vi "Configure Adjacent Channel Power (Measurement Setup).vi"(0 "VISA resource name":refnum<visa-resource-name>, 5 "ACP Carrier Number (1)":i32=1 min=1, 7 "ACP Measurement Method (0:Mod)":i32(ring) items=["Mod", "Total Power", "Inband Channel Bandwidth", "Both Sides", "Number"], 9 "ACP Display Type (0:Carrier)":i32(ring) items=["Carrier", "Offset Channel", "All"], 11 "error in (no error)":errorcluster) -> (4 "VISA resource name out":refnum<visa-resource-name>, 15 "error out":errorcluster)   [LabVIEW 2020, in "Anritsu Signal Analyzer Series.lvlib"]
doc: "Configures the ACP measurement parameters settings of the spectrum analyzer."
uses:
  Anritsu Signal Analyzer Series.lvlib
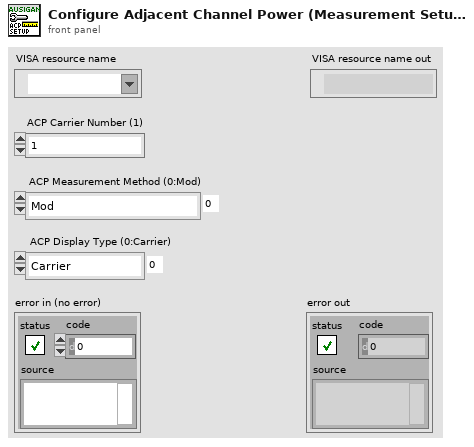
[diagram p1: front panel]
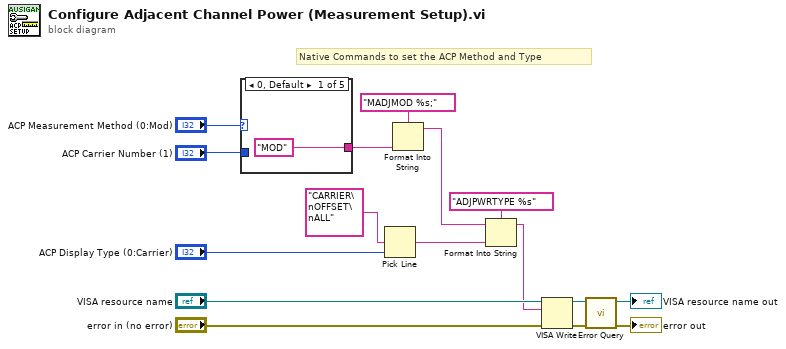
[diagram p0: block diagram]
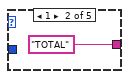
[diagram p2: hidden frame]
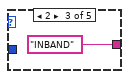
[diagram p3: hidden frame]
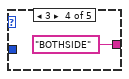
[diagram p4: hidden frame]
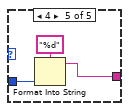
[diagram p5: hidden frame]
diagram:
  # "Native Commands to set the ACP Method and Type"
  n1 = case shown="0, Default" "ACP Measurement Method (0:Mod)" {
    tunnel: ["MOD" ("_Case0") "TOTAL" ("_Case1") "INBAND" ("_Case1") "BOTHSIDE" ("_Case1") w21] -> w9
    tunnel: "ACP Carrier Number (1)" -> [_ _ _ _ w23]
    frame 0, Default {
    }
    frame 1 {
    }
    frame 2 {
    }
    frame 3 {
    }
    frame 4 {
      n2 = Format Into String(format string="%d" ("_Case1"), w23) -> (resulting string=w21:string)  [unwired: 2 in, 1 out]
    }
  }
  n3 = Pick Line(multi-line string="CARRIER\nOFFSET\nALL" ("複数行文字列"), line index="ACP Display Type (0:Carrier)") -> (output string=w2:string)  [unwired: 1 in]
  n4 = Format Into String(format string="MADJMOD %s;" ("_CommandSet"), w9) -> (resulting string=w7:string)  [unwired: 2 in, 1 out]
  n5 = Format Into String(format string="ADJPWRTYPE %s" ("_CommandSet"), initial string=w7, w2) -> (resulting string=w1:string)  [unwired: 1 in, 1 out]
  n6 = VISA Write(VISA resource name="VISA resource name", write buffer=w1, error in (no error)="error in (no error)") -> (VISA resource name out=w4:refnum<visa-resource-name>, error out=w5:errorcluster)  [unwired: 1 out]
  n7 = call "Error Query.vi"("error in (no error)"=w5, "VISA resource name"=w4) -> ("error out"=→"error out":errorcluster, "VISA resource name out"=→"VISA resource name out":refnum<visa-resource-name>)  [unwired: 6 in, 2 out]
